vi "generate_error.vi"(6 "show call chain? (T)":bool=TRUE, 8 "error in (no error)":errorcluster, 10 "data":variant, 11 "error":T1) -> (0 "error out":errorcluster)   [LabVIEW 2015, in "lv-bin-plink.lvlib"]
uses:
  lv-bin-plink.lvlib
  _controls/error.ctl
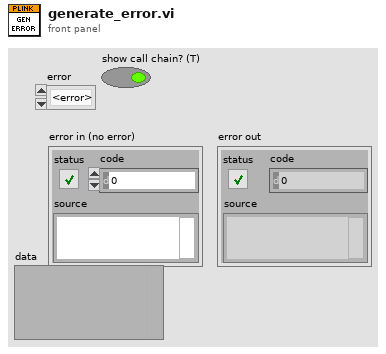
[diagram p1: front panel]
types:
  T1 = typedef "lv-bin-plink.lvlib/error.ctl" = enum16{"<error>", "bad_configuration", "standard_error", "plink_x86_missing", "plink_x64_missing"}
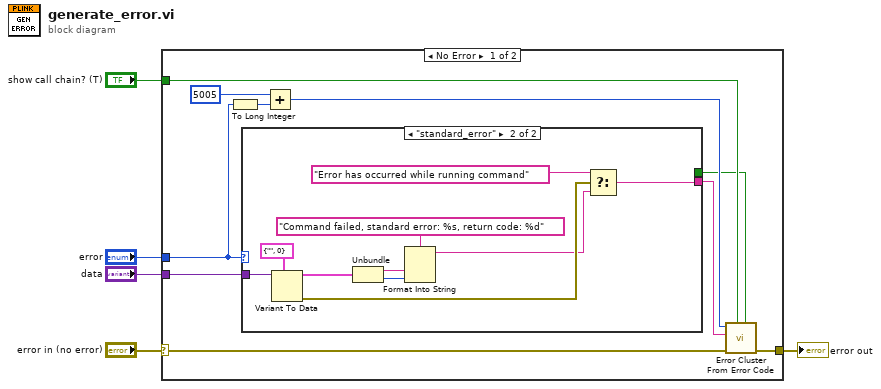
[diagram p0: block diagram]
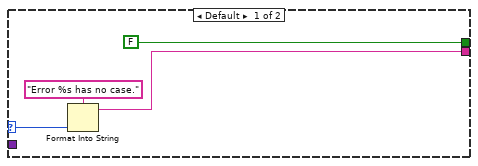
[diagram p2: hidden frame]
diagram:
  n1 = case shown="No Error" "error in (no error)" {
    selector: "error in (no error)" -> [w10 w30]
    tunnel: "data" -> [w9 _]
    tunnel: [w15 w30] -> w3
    tunnel: "error" -> [w8 _]
    tunnel: "show call chain? (T)" -> [w11 _]
    frame No Error {
      n2 = To Long Integer(number=w8) -> (32bit integer=w13:i32)
      n3 = case shown="\"standard_error\"" w8 {
        selector: w8 -> [w18 _]
        tunnel: w9 -> [_ w29]
        tunnel: [w17 w21] -> w6
        tunnel: [FALSE _] -> w7
        frame Default {
          n4 = Format Into String(format string="Error %s has no case.", w18) -> (resulting string=w17:string)  [unwired: 2 in, 1 out]
        }
        frame "standard_error" {
          n5 = Variant To Data(type=cluster{string, "return code":i32} {"", "return code"=0} ("cluster"), Variant=w29) -> (data=w27:cluster{string, "return code":i32}, error out=w26:errorcluster)  [unwired: 1 in]
          n6 = Unbundle(w27) -> (w25:string, "return code"=w24:i32)
          n7 = Format Into String(format string="Command failed, standard error: %s, return code: %d", w25, w24) -> (resulting string=w23:string)  [unwired: 2 in, 1 out]
          n8 = Select(t="Error has occurred while running command", s=w26, f=w23) -> (s? t:f=w21:string)
        }
      }
      n9 = Add(x=5005, y=w13) -> (x+y=w12:i32)
      n10 = call <vilib>:"Error Cluster From Error Code.vi"("is warning? (False)"=w7, "show call chain? (False)"=w11, "error in (no error)"=w10, "error message (\"\")"=w6, "error code (0)"=w12) -> ("error out"=w15:errorcluster)  [unwired: 4 in]
    }
    frame Error {
    }
  }
  "error out" <- w3
